vi "XIPIN_CPRI_8_5.vi"   [LabVIEW 2017]
doc: "The Xilinx CPRI core is a fully tested layer 1 and layer 2 implementation designed to CPRI specification v6.0. An example design and development scripts are provided to ease development of a customized, fully compliant system.\n------------------------------------\n<b>Need License</b> : Yes\n<b>Interface</b> : AXI4 AXI4-Stream"
uses:
  <vilib>/rvi/XilinxIP/XIPIN_XNode/niFpgaXIPIN.xnode
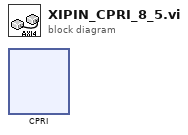
[diagram p0: block diagram]
diagram:
  n1 = xnode ("CPRI")() -> ()
